vi "createArrayToLog.vi"(1 "cluster_select":cluster{"Label.Text":string, bool}[](array[cluster]), 2 "Controls[]":refnum<vi>[](array[refnum])) -> (0 "array_to_log":dbl[](array[numeric]))   [LabVIEW 2021]
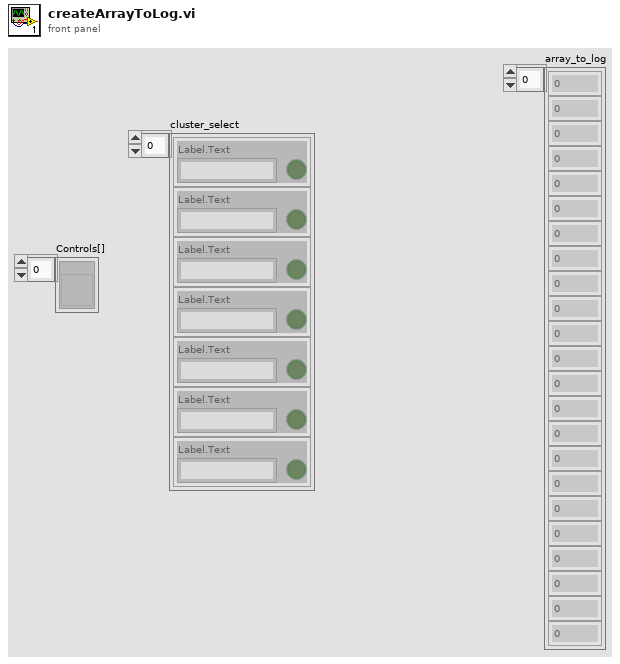
[diagram p1: front panel]
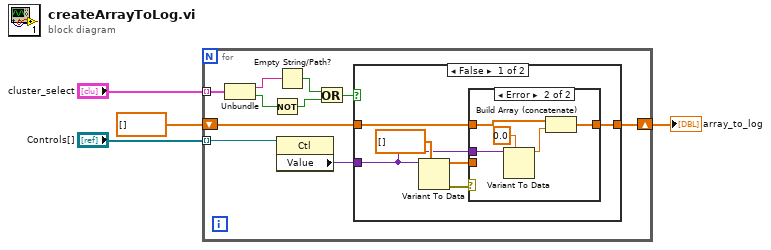
[diagram p0: block diagram]
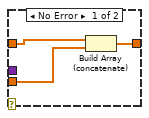
[diagram p2: hidden frame]
diagram:
  n1 = for {
    tunnel: "cluster_select" -> [w9] mode=indexing
    tunnel: "Controls[]" -> [w8] mode=indexing
    shift-right: [w5] -> w2
    shift-left: dbl[] [] -> [w6]
    n2 = Unbundle(w9) -> ("Label.Text"=w13:string, w11:bool)
    n3 = Not(x=w11) -> (.not. x?=w12:bool)
    n4 = Empty String/Path?(string/path=w13) -> (empty?=w10:bool)
    n5 = property class="Ctl"(reference=w8) -> ("Value"=w7:variant)  [unwired: 1 in, 2 out]
    n6 = Or(x=w10, y=w12) -> (x .or. y?=w14:bool)
    n7 = case shown="False" w14 {
      tunnel: w7 -> [w18 _]
      tunnel: [w16 w29] -> w5
      tunnel: w6 -> [w17 w29]
      frame False {
        n8 = Variant To Data(type=dbl[] [], Variant=w18) -> (data=w15:dbl[], error out=w19:errorcluster)  [unwired: 1 in]
        n9 = case shown="Error" w19 {
          tunnel: w18 -> [_ w27]
          tunnel: w17 -> [w22 w25]
          tunnel: [w21 w24] -> w16
          tunnel: w15 -> [w23 _]
          frame No Error {
            n10 = Build Array (concatenate)(w22, w23) -> (w21:dbl[])
          }
          frame Error {
            n11 = Variant To Data(type=0.0, Variant=w27) -> (data=w26:dbl)  [unwired: 1 in, 1 out]
            n12 = Build Array (concatenate)(w25, w26) -> (w24:dbl[])
          }
        }
      }
      frame True {
      }
    }
  }
  "array_to_log" <- w2
